vi "Enable_Disable a Motor.vi"(8 "error in (no error)":errorcluster, 9 "enable/disable":bool, 10 "Index":i32, 11 "Motions in":refnum<class "Motions.lvclass">) -> (0 "error out":errorcluster, 3 "Motions out":refnum<class "Motions.lvclass">)   [LabVIEW 2016, in "Hardware.lvlib" / "Motions.lvlib" / "Motions.lvclass"]
uses:
  <userlib>/Common Components/Hardware/Abstract System/Motions/Motions/Motions.lvclass
  <userlib>/Common Components/Hardware/Abstract System/Motions/Motions/Data_Index.ctl
  <vilib>/addons/_JKI.lib/Serialization/JSON/JKI JSON Serialization.lvlib
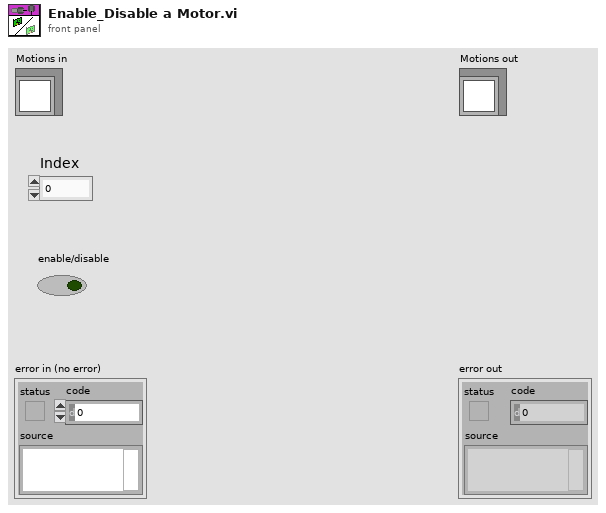
[diagram p1: front panel]
types:
  T1 = typedef "Hardware.lvlib/Motions.lvlib/Motions.lvclass/Data_Index.ctl" = cluster{"Index":i32}
  T2 = cluster{"Action Name":string, "Action Data":string}
  T3 = cluster{"Action Name":string, "Action Data":string}[]
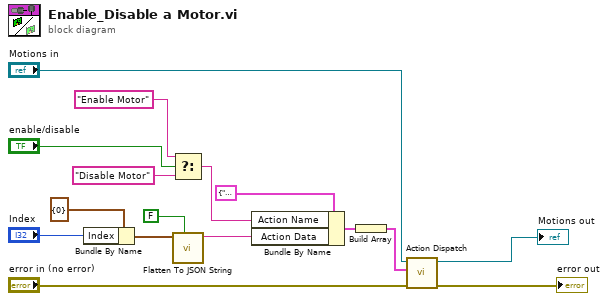
[diagram p0: block diagram]
diagram:
  n1 = Bundle By Name(cluster=T1 {"Index"=0} ("Move Data cluster"), "Index"="Index") -> (w11:T1)
  n2 = Select(t="Enable Motor", s="enable/disable", f="Disable Motor") -> (s? t:f=w13:string)
  n3 = call <vilib>:"Flatten To JSON String.vi"("Multiline (T)"=FALSE, "Variant"=w11) -> ("JSON String"=w10:string)  [unwired: 8 in, 1 out]
  n4 = Bundle By Name(cluster=T2 {"Action Name"="", "Action Data"=""} ("Action"), "Action Name"=w13, "Action Data"=w10) -> (w9:T2)
  n5 = Build Array(w9) -> (w8:T3)
  n6 = call <userlib>:"Action Dispatch.vi"("error in (no error)"="error in (no error)", "Actions"=w8, "Motions in"="Motions in") -> ("error out"=→"error out":errorcluster, "Motions out"=→"Motions out":refnum<class "Motions.lvclass">)  [unwired: 7 in]
